vi "Modbus Read PLC Registers.vi"(8 "error in (no error)":errorcluster, 11 "Modbus Master in":refnum<class "Modbus Master.lvclass">) -> (0 "error out":errorcluster, 2 "Input Registers":u16[](array[numeric]), 3 "Modbus Master out":refnum<class "Modbus Master.lvclass">)   [LabVIEW 2020, in "Modbus.lvlib"]
uses:
  Modbus.lvlib
  <vilib>/NI/Modbus Library/API/Master/Modbus Master.lvclass
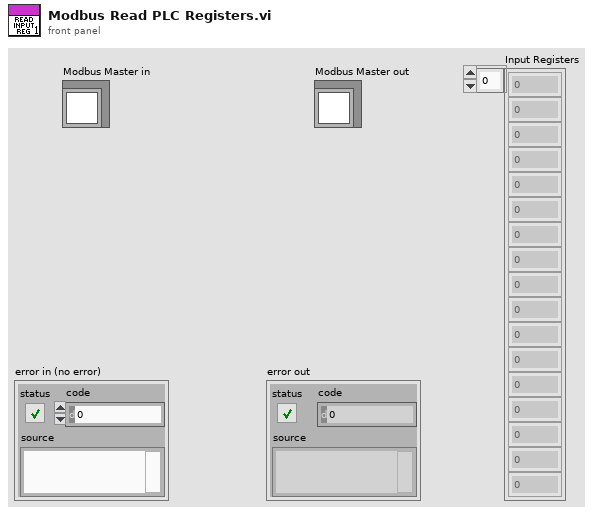
[diagram p1: front panel]
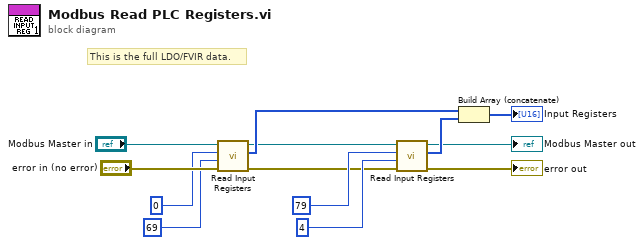
[diagram p0: block diagram]
diagram:
  # "This is the full LDO/FVIR data."
  n1 = call-dynamic "Read Input Registers.vi"("error in"="error in (no error)", "number of inputs"=u16 69, "starting address"=u16 0, "Modbus master in"="Modbus Master in") -> ("error out"=w5:errorcluster, "register values"=w12:u16[], "Modbus master out"=w7:refnum<class "Modbus Master.lvclass">)  [unwired: 5 in]
  n2 = call-dynamic "Read Input Registers.vi"("error in"=w5, "number of inputs"=u16 4, "starting address"=u16 79, "Modbus master in"=w7) -> ("error out"=→"error out":errorcluster, "register values"=w11:u16[], "Modbus master out"=→"Modbus Master out":refnum<class "Modbus Master.lvclass">)  [unwired: 5 in]
  n3 = Build Array (concatenate)(w12, w11) -> (→"Input Registers":u16[])
